vi "Output on.vi"(8 "error in (no error)":errorcluster, 10 "Output On":bool, 11 "Keithley 24xx in":refnum<class "Keithley 24xx.lvclass">) -> (0 "error out":errorcluster, 3 "Keithley 24xx out":refnum<class "Keithley 24xx.lvclass">)   [LabVIEW 2020, in "Keithley 24xx.lvclass"]
uses:
  Keithley 24xx.lvclass
  C:/Sandbox/Git_Sandbox/WiSpry Test Framework source code (LV20)/WiSpry Test Framework/Instruments/Instrument.lvclass
  Instrument.lvclass/Instrument.ctl
  Instrument.lvclass
  <instrlib>/Keithley 24XX/Keithley 24XX.lvlib
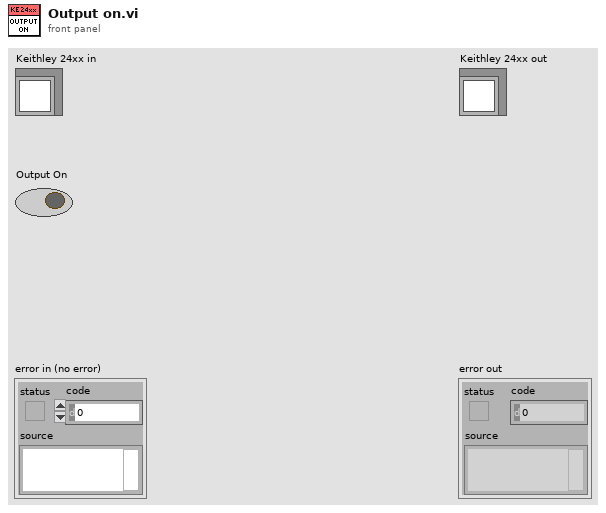
[diagram p1: front panel]
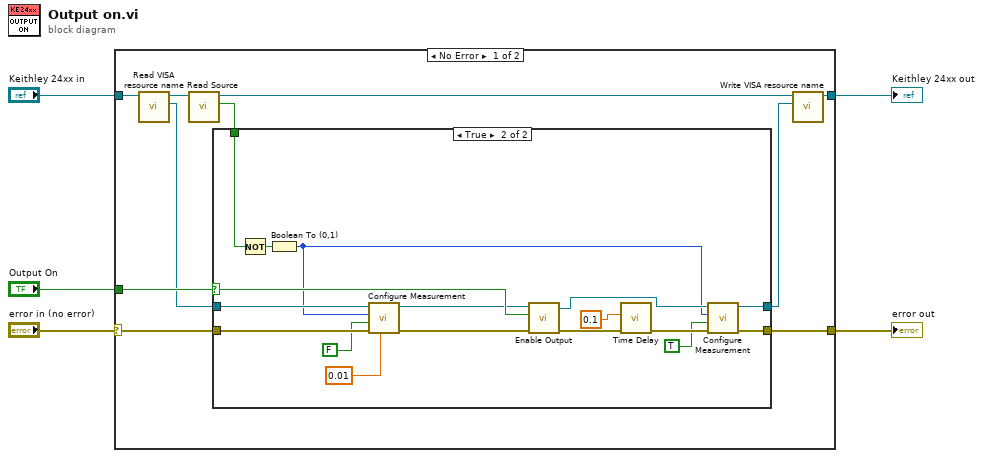
[diagram p0: block diagram]
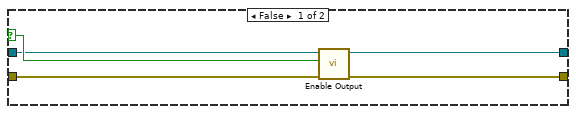
[diagram p2: hidden frame]
diagram:
  n1 = case shown="No Error" "error in (no error)" {
    selector: "error in (no error)" -> [w8 w39]
    tunnel: [w11 w39] -> w5
    tunnel: [w14 w38] -> w4
    tunnel: "Output On" -> [w13 _]
    tunnel: "Keithley 24xx in" -> [w15 w38]
    frame No Error {
      n2 = call "Read VISA resource name.vi"("Instrument in"=w15) -> ("VISA resource name"=w10:refnum<visa-resource-name>, "Instrument out"=w7:refnum<class "Keithley 24xx.lvclass">)  [unwired: 9 in]
      n3 = call-dynamic "Read Source.vi"("Power Supply in"=w7) -> ("Source"=w9:bool, "Power Supply out"=w6:refnum<class "Keithley 24xx.lvclass">)  [unwired: 9 in]
      n4 = case shown="True" w13 {
        selector: w13 -> [w19 w37]
        tunnel: [w16 w28] -> w12
        tunnel: [w17 w29] -> w11
        tunnel: w10 -> [w18 w25]
        tunnel: w9 -> [_ w34]
        tunnel: w8 -> [w20 w32]
        frame False {
          n5 = call <instrlib>:"Enable Output.vi"("error in (no error)"=w20, "Enable Output (T: Enable)"=w19, "VISA resource name"=w18) -> ("error out"=w17:errorcluster, "VISA resource name out"=w16:refnum<visa-resource-name>)  [unwired: 7 in]
        }
        frame True {
          n6 = Not(x=w34) -> (.not. x?=w33:bool)
          n7 = Boolean To (0,1)(Boolean=w33) -> (0, 1=w21:i16)
          n8 = call <instrlib>:"Configure Measurement.vi"("Manual Range (1.0)"=0.01, "error in (no error)"=w32, "Enable Auto Range (T:Enable)"=FALSE, "Function (0: Volts)"=w21, "VISA resource name"=w25) -> ("error out"=w31:errorcluster, "VISA resource name out"=w26:refnum<visa-resource-name>)  [unwired: 5 in]
          n9 = call <instrlib>:"Enable Output.vi"("error in (no error)"=w31, "Enable Output (T: Enable)"=w37, "VISA resource name"=w26) -> ("error out"=w36:errorcluster, "VISA resource name out"=w27:refnum<visa-resource-name>)  [unwired: 7 in]
          n10 = call "Time Delay"("error in (no error)"=w36, "Delay Time (s)"=0.1) -> ("error out"=w30:errorcluster)  [unwired: 9 in]
          n11 = call <instrlib>:"Configure Measurement.vi"("error in (no error)"=w30, "Enable Auto Range (T:Enable)"=TRUE, "Function (0: Volts)"=w21, "VISA resource name"=w27) -> ("error out"=w29:errorcluster, "VISA resource name out"=w28:refnum<visa-resource-name>)  [unwired: 6 in]
        }
      }
      n12 = call "Write VISA resource name.vi"("VISA resource name"=w12, "Instrument in"=w6) -> ("Instrument out"=w14:refnum<class "Keithley 24xx.lvclass">)  [unwired: 9 in]
    }
    frame Error {
    }
  }
  "error out" <- w5
  "Keithley 24xx out" <- w4
